vi "bh3_set_accelerometer_packet_transmit_state.vi"(7 "enable?":bool, 8 "error in (no error)":errorcluster, 11 "bt connection ID in":refnum<k31>) -> (0 "error out":errorcluster, 3 "bt connection ID out":refnum<k31>)   [LabVIEW 2013]
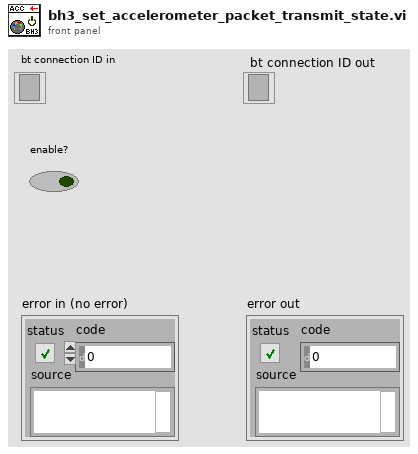
[diagram p1: front panel]
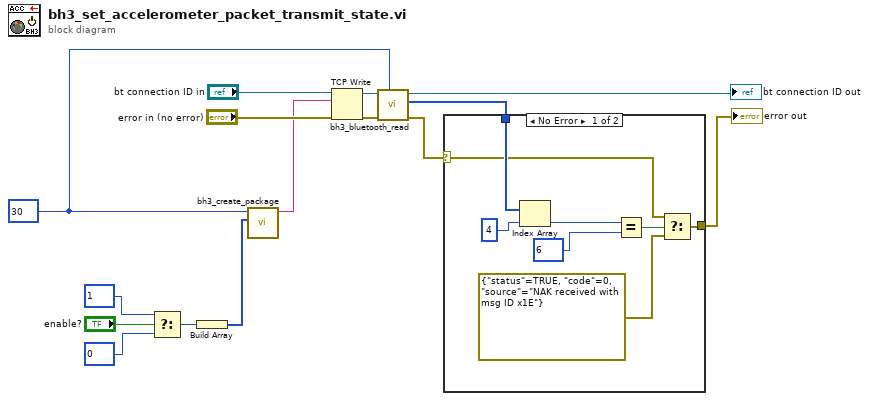
[diagram p0: block diagram]
diagram:
  w1 = u8 30 ("msg_ID")
  n1 = Select(t=u8 1 ("msg_ID"), s="enable?", f=u8 0 ("msg_ID")) -> (s? t:f=w9:u8)
  n2 = Build Array(w9) -> (w8:u8[])
  n3 = call "bh3_create_package.vi"("Payload"=w8, "msg_ID"=w1) -> ("package string"=w13:string)  [unwired: 8 in, 1 out]
  n4 = TCP Write(connection ID="bt connection ID in", data in=w13, error in (no error)="error in (no error)") -> (connection ID out=w5:refnum<k31>, error out=w7:errorcluster)  [unwired: 1 in, 1 out]
  n5 = call "bh3_bluetooth_read.vi"("command_expected(x00)"=w1, "error in (no error)"=w7, "bt connection ID in"=w5) -> ("error out"=w2:errorcluster, "response byte array"=w4:u8[], "bt connection ID out"=→"bt connection ID out":refnum<k31>)  [unwired: 6 in]
  n6 = case shown="No Error" w2 {
    selector: w2 -> [w16 w24]
    tunnel: w4 -> [w23 _]
    tunnel: [w18 w24] -> w3
    frame No Error {
      n7 = Index Array(array=w23, index=4) -> (element=w21:u8)
      n8 = Equal?(x=w21, y=u8 6 ("msg_ID")) -> (x = y?=w19:bool)
      n9 = Select(t=w16, s=w19, f=errorcluster {"status"=TRUE, "code"=0, "source"="NAK received with msg ID x1E"} ("s? t:f")) -> (s? t:f=w18:errorcluster)
    }
    frame Error {
    }
  }
  "error out" <- w3
